vi "SVT Human Vibration Weighting Filter (Fixed Rates) (1 Ch).vi"(6 "reset filter (F)":bool, 8 "error in (no error)":errorcluster, 10 "weighting":u16(ring) items=["Linear"=0, "Wh: hand-arm"=13, "Wb: vertical whole-body"=8, "Wc: horizontal whole-body"=9, "Wd: horizontal whole-body"=10, "We: rotational whole-body"=11, "Wj: vertical head"=14, "Wk: vertical whole-body"=15, "Wm: whole-body in buildings"=16, "Wf: low-frequency whole-body"=12], 11 "scaled signal [EU]":waveform(dbl)) -> (0 "error out":errorcluster, 3 "weighted signal [EU]":waveform(dbl))   [LabVIEW 2017, in "SoundVib_HumanVibration.lvlib"]
doc: "Applies the selected human vibration weighting to a scaled signal expressed in engineering units. This VI complies with ISO 8041:2005 (E), JIS B 7760:2004, and JISB 7761:2004 standards. Each instance of this VI maintains its own state; use the N Channel instance of this VI to process an array of channels. This VI operates on time-continuous data; it resets on a discontinuity. Wire data to the <B>scaled signal [EU]</B> input to determine the polymorphic instance to use or manually select the instance."
uses:
  <vilib>/addons/Sound and Vibration/svt_Weighting/SoundVib_HumanVibration.lvlib
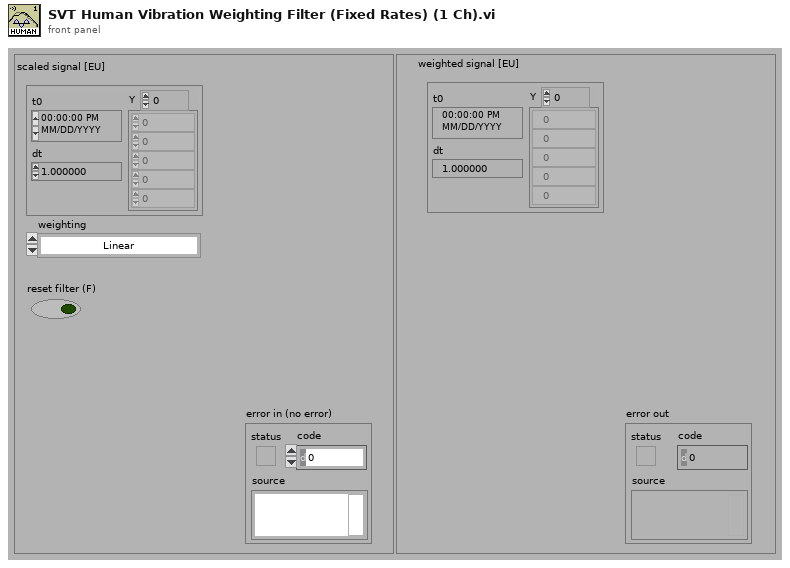
[diagram p1: front panel]
types:
  T1 = typedef "svc_Weighting Filter Text Ring.ctl" = u16
  T2 = cluster{"filter structure":enum32{"IIR 2nd Order", "IIR 4th Order"}, "Reverse Coefficients":dbl[], "Forward Coefficients":dbl[]}
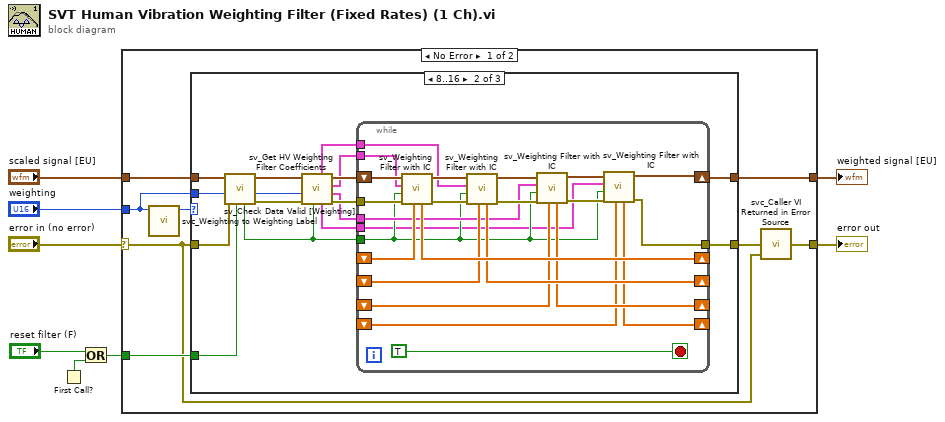
[diagram p0: block diagram]
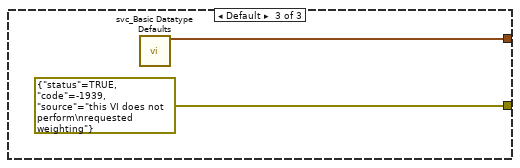
[diagram p3: hidden frame]
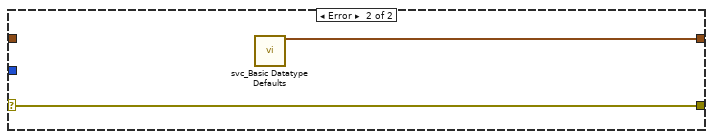
[diagram p4: hidden frame]
diagram:
  n1 = First Call?() -> (First Call?: T/F=w1:bool)
  n2 = Or(x="reset filter (F)", y=w1) -> (x .or. y?=w5:bool)
  n3 = case shown="No Error" "error in (no error)" {
    selector: "error in (no error)" -> [w9 w62]
    tunnel: [w13 w62] -> w8
    tunnel: [w16 w61] -> w7
    tunnel: "scaled signal [EU]" -> [w15 _]
    tunnel: w5 -> [w14 _]
    tunnel: "weighting" -> [w10 _]
    frame No Error {
      n4 = call <vilib>:"svc_Weighting to Weighting Label.vi"("weighting filter"=w10) -> ("weighting enum"=w11:T1)  [unwired: 9 in, 1 out]
      n5 = case shown="8..16" w11 {
        tunnel: [w17 w30 errorcluster {"status"=TRUE, "code"=-1939, "source"="this VI does not perform\nrequested weighting"} ("error out")] -> w12
        tunnel: [w18 w34 w60] -> w16
        tunnel: w15 -> [w18 w33 _]
        tunnel: w9 -> [w17 w32 _]
        tunnel: w14 -> [_ w31 _]
        tunnel: w10 -> [_ w29 _]
        frame 0 {
          # "if (weighting == Linear )\nSkip weighting()"
        }
        frame 8..16 {
          n6 = call <vilib>:"sv_Check Data Valid [Weighting].vi"("reset (in)"=w31, "error in (no error)"=w32, "weighting"=w29, "signal in [X]"=w33) -> ("error out"=w26:errorcluster, "weighting"=w27:T1, "signal out [X]"=w28:waveform(dbl), "reset (out)"=w25:bool)  [unwired: 4 in]
          n7 = call <vilib>:"sv_Get HV Weighting Filter Coefficients.vi"("reset filter (F)"=w25, "error in (no error)"=w26, "weighting filter"=w27, "scaled signal"=w28) -> ("error out"=w23:errorcluster, "a-v filter coefficients"=w20:T2, "LP filter coefficients"=w21:T2, "dup scaled signal"=w24:waveform(dbl), "upward step filter coefficients"=w19:T2, "HP filter coefficients"=w22:T2)  [unwired: 2 in]
          n8 = while {
            shift-left: _ -> [w57]
            shift-right: [w56] -> _
            tunnel: w25 -> [w40]
            tunnel: [w48] -> w30
            tunnel: w23 -> [w54]
            shift-right: [w37] -> w34
            shift-left: w24 -> [w55]
            shift-right: [w46] -> _
            shift-left: _ -> [w47]
            shift-right: [w45] -> _
            shift-left: _ -> [w44]
            shift-right: [w43] -> _
            shift-left: _ -> [w42]
            tunnel: w22 -> [w35]
            tunnel: w21 -> [w36]
            tunnel: w20 -> [w41]
            tunnel: w19 -> [w39]
            stop <- TRUE stop-if-true
            n9 = call <vilib>:"sv_Weighting Filter with IC.vi"("Initial Filter State"=w57, "error in (no error)"=w54, "reset filter (F)"=w40, "filter coefficients"=w36, "signal [V]"=w55) -> ("error out"=w50:errorcluster, "filtered signal [EU]"=w49:waveform(dbl), "Final Filter State"=w56:dbl[])  [unwired: 4 in]
            n10 = call <vilib>:"sv_Weighting Filter with IC.vi"("Initial Filter State"=w47, "error in (no error)"=w50, "reset filter (F)"=w40, "filter coefficients"=w35, "signal [V]"=w49) -> ("error out"=w53:errorcluster, "filtered signal [EU]"=w52:waveform(dbl), "Final Filter State"=w46:dbl[])  [unwired: 4 in]
            n11 = call <vilib>:"sv_Weighting Filter with IC.vi"("Initial Filter State"=w44, "error in (no error)"=w53, "reset filter (F)"=w40, "filter coefficients"=w41, "signal [V]"=w52) -> ("error out"=w51:errorcluster, "filtered signal [EU]"=w38:waveform(dbl), "Final Filter State"=w45:dbl[])  [unwired: 4 in]
            n12 = call <vilib>:"sv_Weighting Filter with IC.vi"("Initial Filter State"=w42, "error in (no error)"=w51, "reset filter (F)"=w40, "filter coefficients"=w39, "signal [V]"=w38) -> ("error out"=w48:errorcluster, "filtered signal [EU]"=w37:waveform(dbl), "Final Filter State"=w43:dbl[])  [unwired: 4 in]
          }
        }
        frame Default {
          n13 = call <vilib>:"svc_Basic Datatype Defaults.vi"() -> ("empty waveform"=w60:waveform(dbl))  [unwired: 7 in, 12 out]
        }
      }
      n14 = call <vilib>:"svc_Caller VI Returned in Error Source.vi"("warning input to caller"=w9, "error in (no error)"=w12) -> ("error out"=w13:errorcluster)  [unwired: 3 in]
    }
    frame Error {
      n15 = call <vilib>:"svc_Basic Datatype Defaults.vi"() -> ("empty waveform"=w61:waveform(dbl))  [unwired: 7 in, 12 out]
    }
  }
  "error out" <- w8
  "weighted signal [EU]" <- w7
